vi "SPCC_Assignment_Server.vi"() -> ()   [LabVIEW 2023]
uses:
  LoginEnumStates.ctl
  <vilib>/Utility/file.llb/Write Delimited Spreadsheet (string).vi
  <vilib>/Utility/file.llb/Read Delimited Spreadsheet (string).vi
  <vilib>/regexp/Match Regular Expression.xnode
panel:
  in  "LoginUI":enum32{"Page 1"}(tab)
  in  "Password":string
  in  "User Name":string
  in  "btnLogin":bool
  in  "ZoneUI":enum32{"Page 1"}(tab)
  out "date/time string":string
  out "Alert":bool
  out "1T":bool caption="1A 3"
  out "1B":bool caption="1A 2"
  out "1A":bool
  out "Zone1":bool
  out "6T":bool caption="1A 3"
  out "6B":bool caption="1A 2"
  out "6A":bool caption="1A"
  out "Zone6":bool
  out "5T":bool caption="1A 3"
  out "5B":bool caption="1A 2"
  out "5A":bool caption="1A"
  out "Zone5":bool
  out "4T":bool caption="1A 3"
  out "4B":bool caption="1A 2"
  out "4A":bool caption="1A"
  out "Zone4":bool
  out "3T":bool caption="1A 3"
  out "3B":bool caption="1A 2"
  out "3A":bool caption="1A"
  out "Zone3":bool
  out "2T":bool caption="1A 3"
  out "2B":bool caption="1A 2"
  out "2A":bool caption="1A"
  out "Zone2":bool
  out "UserType":string
  in  "UserUi":enum32{"Page 1"}(tab)
  in  "btnUserEnd":bool
  in  "btnUserLogout":bool
  in  "AdminUI":enum32{"Page 2"}(tab)
  in  "btnViewLogs":bool
  in  "btnRegister":bool
  in  "btnAdminLogout":bool
  in  "btnAdminEnd":bool
  in  "User Table":string[][](table)
  in  "Tamper":cluster{u32, u32}[](array[cluster])
  in  "Bypass":cluster{u32, u32}[](array[cluster])
  in  "Alarm":cluster{u32, u32}[](array[cluster])
  in  "Normal":cluster{u32, u32}[](array[cluster])
  in  "ViewLogsUI":enum32{"Page 1"}(tab)
  in  "LogsTable":string[][](table)
  in  "btnMainMenu":bool
  # "LOGIN"
  # "Green   = Normal\nRed       = Alarm\nBlue      = Bypass\nOrange = Tamper"
  # "Zone Status Indicator"
  # "Zone 1"
  # "Alarm"
  # "Bypass"
  # "Tamper"
  # "Zone 6"
  # "Alarm"
  # "Bypass"
  # "Tamper"
  # "Zone 5"
  # "Alarm"
  # "Bypass"
  # "Tamper"
  # "Zone 4"
  # "Alarm"
  # "Bypass"
  # "Tamper"
  # "Zone 3"
  # "Alarm"
  # "Bypass"
  # "Tamper"
  # "Zone 2"
  # "Alarm"
  # "Bypass"
  # "Tamper"
  # "ADMIN MENU"
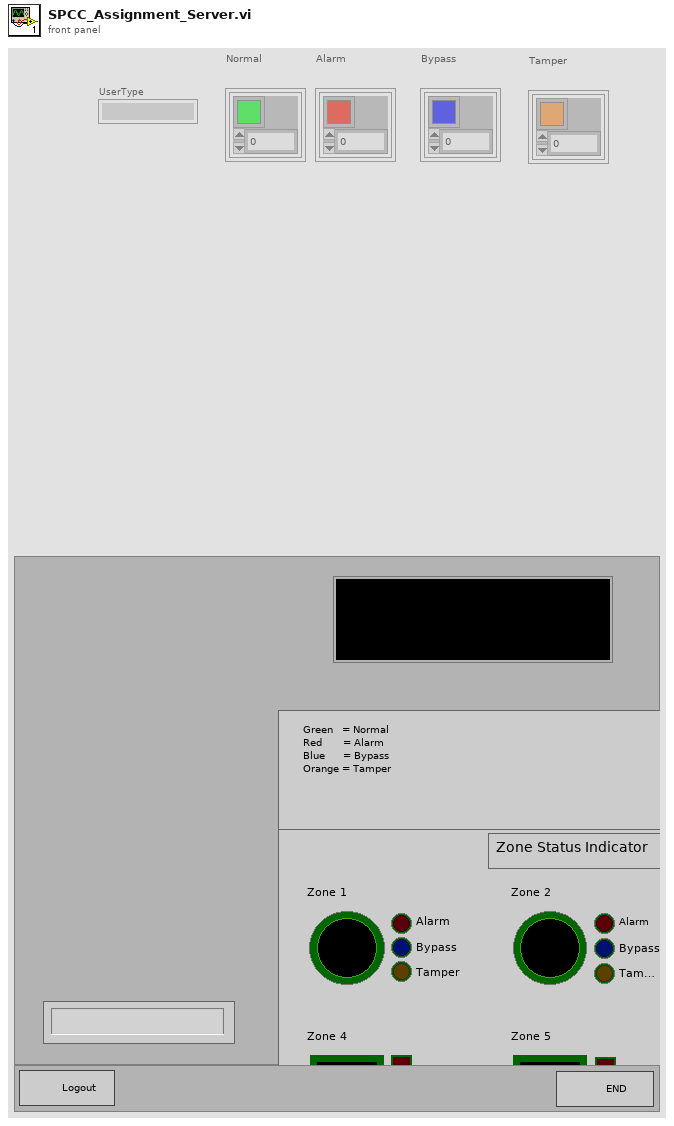
[diagram p1: front panel]
types:
  T1 = typedef "LoginEnumStates.ctl" = enum16{"Init", "Wait", "Login", "UIBuild", "Logout", "Register", "End"}
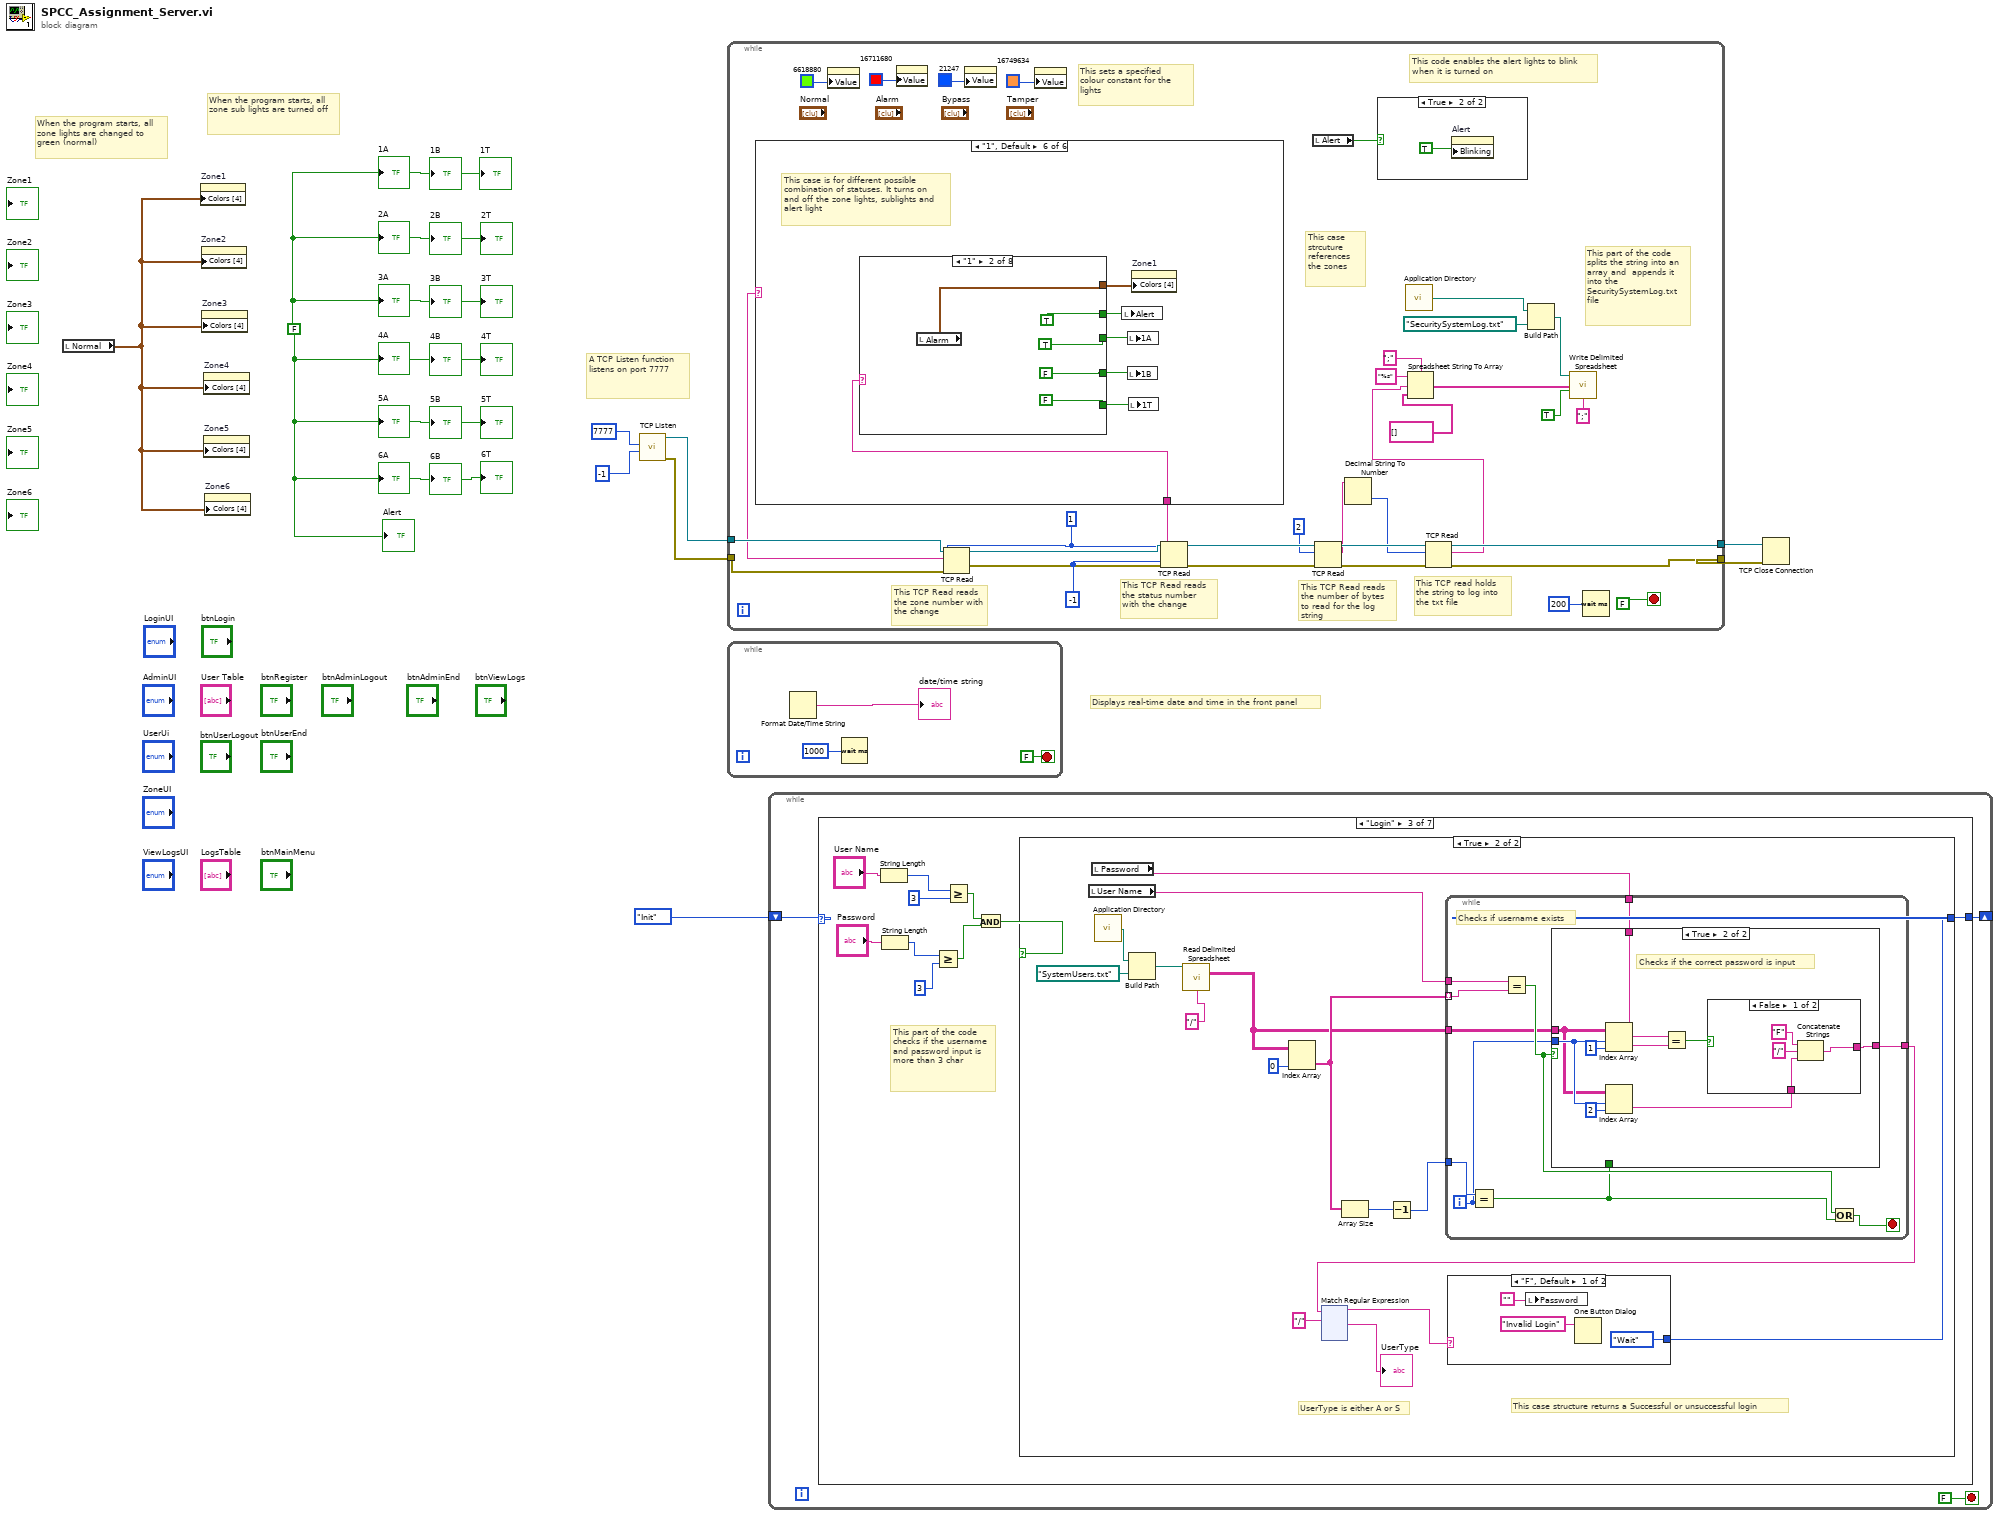
[diagram p0: block diagram]
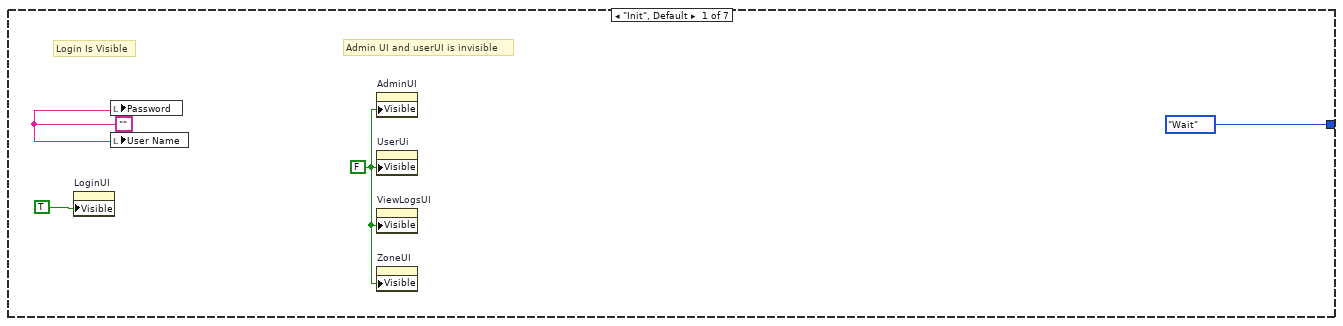
[diagram p2: hidden frame]
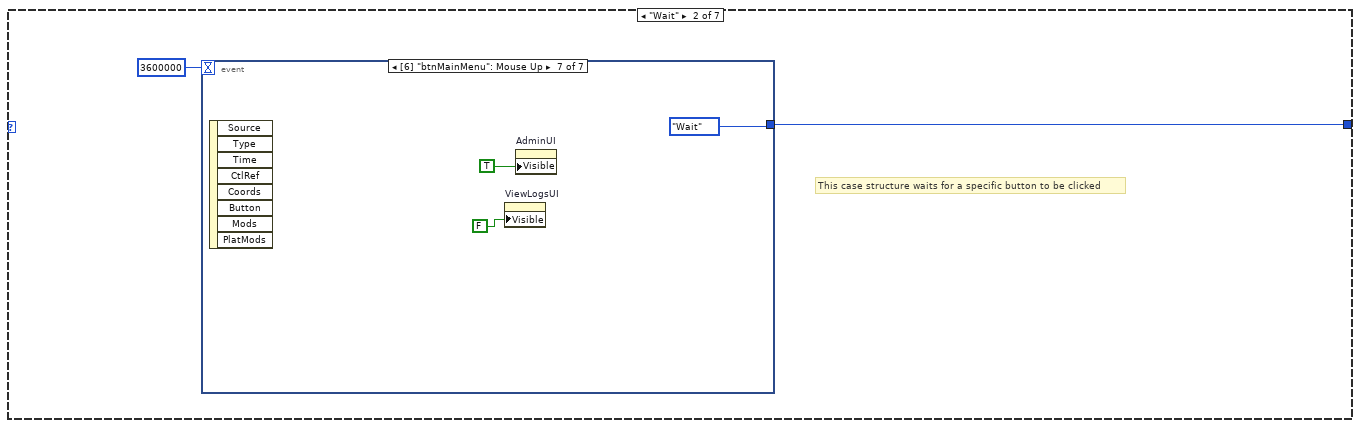
[diagram p3: hidden frame]
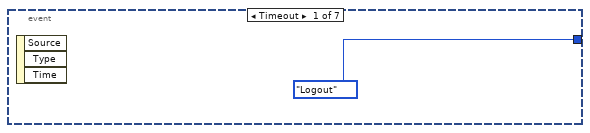
[diagram p4: hidden frame]
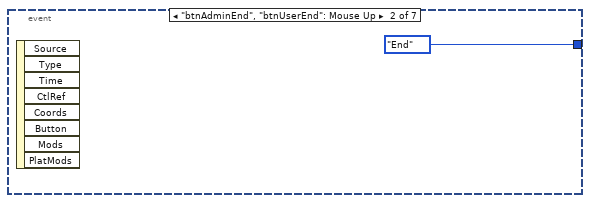
[diagram p5: hidden frame]
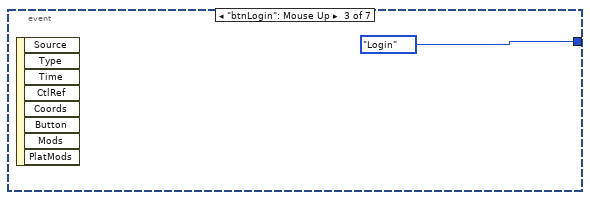
[diagram p6: hidden frame]
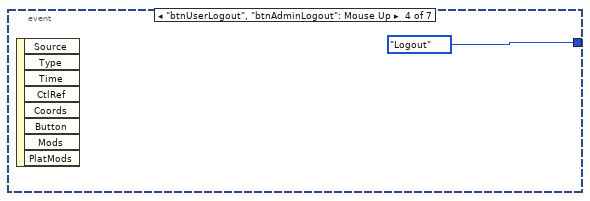
[diagram p7: hidden frame]
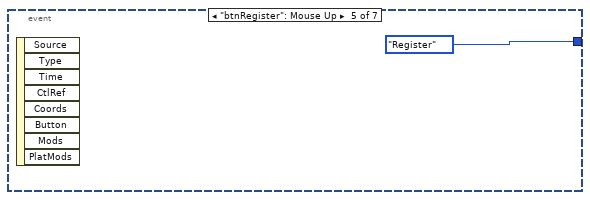
[diagram p8: hidden frame]
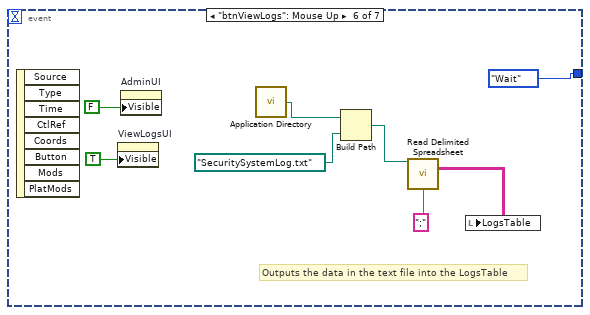
[diagram p9: hidden frame]
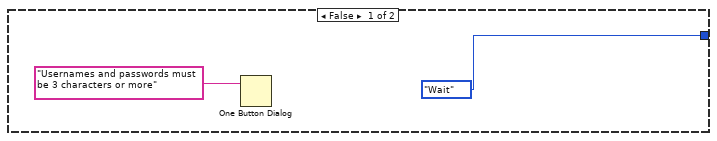
[diagram p10: hidden frame]
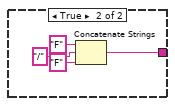
[diagram p12: hidden frame]
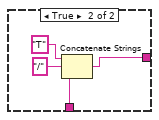
[diagram p13: hidden frame]
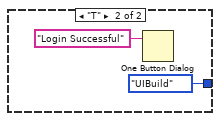
[diagram p14: hidden frame]
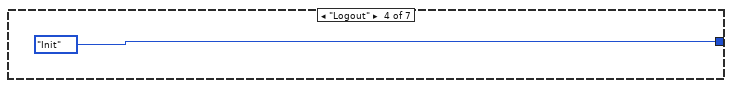
[diagram p15: hidden frame]
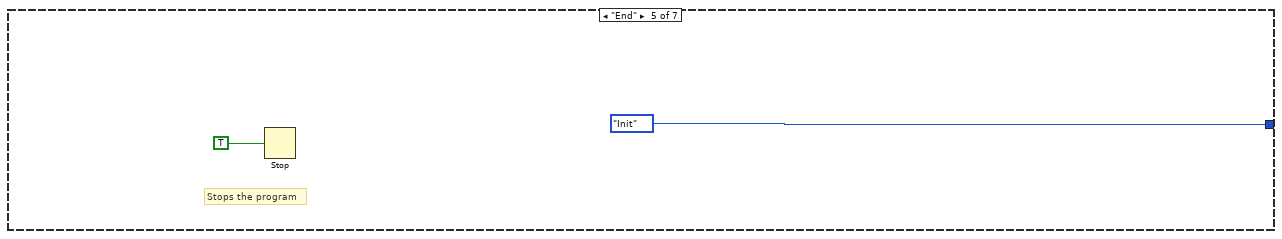
[diagram p16: hidden frame]
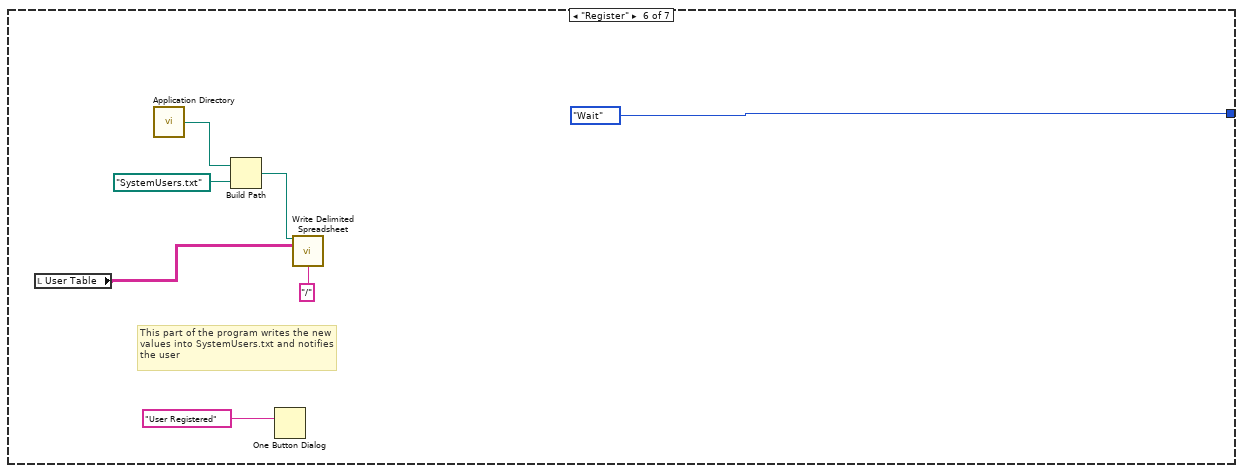
[diagram p17: hidden frame]
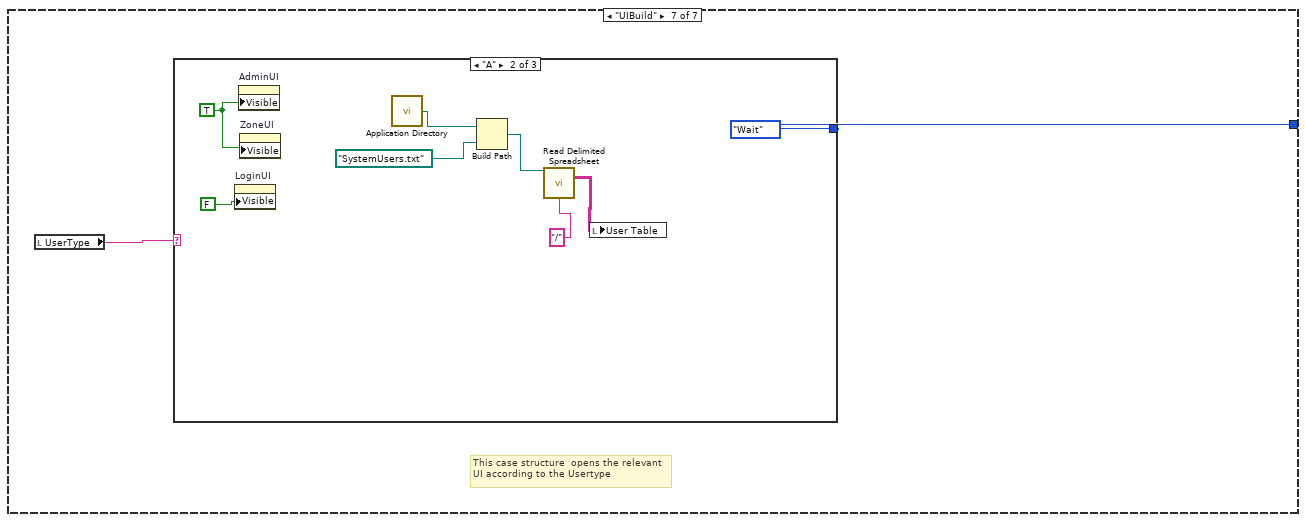
[diagram p18: hidden frame]
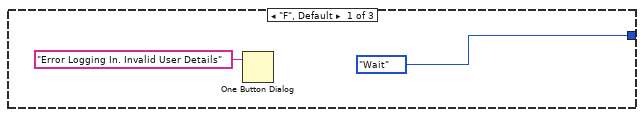
[diagram p19: hidden frame]
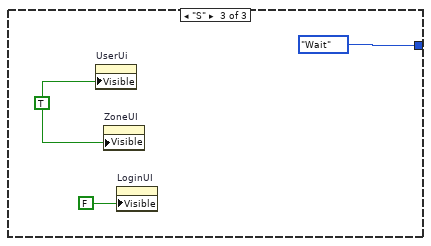
[diagram p20: hidden frame]
diagram:
  w2 = FALSE
  # "Displays real-time date and time in the front panel"
  # "A TCP Listen function listens on port 7777"
  # "When the program starts, all zone sub lights are turned off"
  # "When the program starts, all zone lights are changed to green (normal)"
  n1 = local read "Normal"() -> (w3:cluster{u32, u32}[])
  n2 = property on="Zone1" class="Bool (strict)"("Colors [4]"=w3) -> ()  [unwired: 2 in, 2 out]
  n3 = property on="Zone2" class="Bool (strict)"("Colors [4]"=w3) -> ()  [unwired: 2 in, 2 out]
  n4 = property on="Zone3" class="Bool (strict)"("Colors [4]"=w3) -> ()  [unwired: 2 in, 2 out]
  n5 = property on="Zone4" class="Bool (strict)"("Colors [4]"=w3) -> ()  [unwired: 2 in, 2 out]
  n6 = property on="Zone5" class="Bool (strict)"("Colors [4]"=w3) -> ()  [unwired: 2 in, 2 out]
  n7 = property on="Zone6" class="Bool (strict)"("Colors [4]"=w3) -> ()  [unwired: 2 in, 2 out]
  n8 = call <vilib>:"TCP Listen.vi"("timeout ms (wait forever: -1)"=-1, "port"=u16 7777) -> ("error out"=w7:errorcluster, "connection ID"=w9:refnum<k5>)  [unwired: 5 in, 3 out]
  n9 = while {
    tunnel: w9 -> [w42]
    tunnel: [w30] -> w8
    tunnel: w7 -> [w40]
    tunnel: [w29] -> w6
    stop <- FALSE stop-if-true
    w37 = -1 ("timeout ms (25000)")
    w38 = 1 ("bytes to read")
    # "This case strcuture references the zones"
    # "This sets a specified colour constant for the lights"
    # "This code enables the alert lights to blink when it is turned on"
    # "This part of the code splits the string into an array and  appends it into the SecuritySystemLog.txt file"
    # "This TCP read holds the string to log into the txt file"
    # "This TCP Read reads the number of bytes to read for the log string"
    # "This TCP Read reads the status number with the change"
    # "This TCP Read reads the zone number with the change"
    n10 = property class="ColBox"("Value"=u32 6618880) -> ()  [unwired: 2 in, 2 out]
    n11 = property class="ColBox"("Value"=u32 16711680) -> ()  [unwired: 2 in, 2 out]
    n12 = TCP Read(connection ID=w42, bytes to read=w38, error in (no error)=w40, 9:w37) -> (connection ID out=w41:refnum<k5>, data out=w36:string, error out=w39:errorcluster)  [unwired: 1 in]
    n13 = property class="ColBox"("Value"=u32 21247) -> ()  [unwired: 2 in, 2 out]
    n14 = property class="ColBox"("Value"=u32 16749634) -> ()  [unwired: 2 in, 2 out]
    n15 = TCP Read(connection ID=w41, bytes to read=w38, error in (no error)=w39, 9:w37) -> (connection ID out=w17:refnum<k5>, data out=w43:string, error out=w16:errorcluster)  [unwired: 1 in]
    n16 = case shown="\"1\", Default" w36 {
      tunnel: w43 -> [w51 w90 w131 w171 w210 w251]
      frame "2" {
        # "This case is for different possible combination of statuses. It turns on and off the zone lights, sublights and alert light"
        n17 = case shown="\"0\", Default" w51 {
          tunnel: [w53 w58 w63 w68 w73 w78 w83 w85] -> w50
          tunnel: [w52 TRUE FALSE TRUE FALSE TRUE FALSE w84] -> w49
          tunnel: [w52 FALSE TRUE TRUE FALSE FALSE TRUE w84] -> w48
          tunnel: [w52 FALSE FALSE FALSE TRUE TRUE TRUE w84] -> w47
          tunnel: [w52 TRUE FALSE FALSE TRUE TRUE TRUE w84] -> w46
          frame "0", Default {
            w52 = FALSE
            n18 = local read "Normal"() -> (w53:cluster{u32, u32}[])
          }
          frame "1" {
            n19 = local read "Alarm"() -> (w58:cluster{u32, u32}[])
          }
          frame "2" {
            n20 = local read "Bypass"() -> (w63:cluster{u32, u32}[])
          }
          frame "3" {
            n21 = local read "Bypass"() -> (w68:cluster{u32, u32}[])
          }
          frame "4" {
            n22 = local read "Tamper"() -> (w73:cluster{u32, u32}[])
          }
          frame "5" {
            n23 = local read "Tamper"() -> (w78:cluster{u32, u32}[])
          }
          frame "6" {
            n24 = local read "Tamper"() -> (w83:cluster{u32, u32}[])
          }
          frame "7" {
            w84 = TRUE
            n25 = local read "Tamper"() -> (w85:cluster{u32, u32}[])
          }
        }
        n26 = local write "Alert"(w46) -> ()
        n27 = local write "2A"(w49) -> ()
        n28 = local write "2B"(w48) -> ()
        n29 = local write "2T"(w47) -> ()
        n30 = property on="Zone2" class="Bool (strict)"("Colors [4]"=w50) -> ()  [unwired: 2 in, 2 out]
      }
      frame "3" {
        # "This case is for different possible combination of statuses. It turns on and off the zone lights, sublights and alert light"
        n31 = case shown="\"7\"" w90 {
          tunnel: [w93 w98 w103 w108 w113 w118 w123 w125] -> w91
          tunnel: [w92 TRUE FALSE TRUE FALSE TRUE FALSE w124] -> w89
          tunnel: [w92 FALSE TRUE TRUE FALSE FALSE TRUE w124] -> w88
          tunnel: [w92 FALSE FALSE FALSE TRUE TRUE TRUE w124] -> w87
          tunnel: [w92 TRUE FALSE FALSE TRUE TRUE TRUE w124] -> w86
          frame "0", Default {
            w92 = FALSE
            n32 = local read "Normal"() -> (w93:cluster{u32, u32}[])
          }
          frame "1" {
            n33 = local read "Alarm"() -> (w98:cluster{u32, u32}[])
          }
          frame "2" {
            n34 = local read "Bypass"() -> (w103:cluster{u32, u32}[])
          }
          frame "3" {
            n35 = local read "Bypass"() -> (w108:cluster{u32, u32}[])
          }
          frame "4" {
            n36 = local read "Tamper"() -> (w113:cluster{u32, u32}[])
          }
          frame "5" {
            n37 = local read "Tamper"() -> (w118:cluster{u32, u32}[])
          }
          frame "6" {
            n38 = local read "Tamper"() -> (w123:cluster{u32, u32}[])
          }
          frame "7" {
            w124 = TRUE
            n39 = local read "Tamper"() -> (w125:cluster{u32, u32}[])
          }
        }
        n40 = local write "Alert"(w86) -> ()
        n41 = local write "3A"(w89) -> ()
        n42 = local write "3B"(w88) -> ()
        n43 = local write "3T"(w87) -> ()
        n44 = property on="Zone3" class="Bool (strict)"("Colors [4]"=w91) -> ()  [unwired: 2 in, 2 out]
      }
      frame "4" {
        # "This case is for different possible combination of statuses. It turns on and off the zone lights, sublights and alert light"
        n45 = case shown="\"7\"" w131 {
          tunnel: [w133 w138 w143 w148 w153 w158 w163 w165] -> w130
          tunnel: [w132 TRUE FALSE TRUE FALSE TRUE FALSE w164] -> w129
          tunnel: [w132 FALSE FALSE FALSE TRUE TRUE TRUE w164] -> w128
          tunnel: [w132 FALSE TRUE TRUE FALSE FALSE TRUE w164] -> w127
          tunnel: [w132 TRUE FALSE FALSE TRUE TRUE TRUE w164] -> w126
          frame "0", Default {
            w132 = FALSE
            n46 = local read "Normal"() -> (w133:cluster{u32, u32}[])
          }
          frame "1" {
            n47 = local read "Alarm"() -> (w138:cluster{u32, u32}[])
          }
          frame "2" {
            n48 = local read "Bypass"() -> (w143:cluster{u32, u32}[])
          }
          frame "3" {
            n49 = local read "Bypass"() -> (w148:cluster{u32, u32}[])
          }
          frame "4" {
            n50 = local read "Tamper"() -> (w153:cluster{u32, u32}[])
          }
          frame "5" {
            n51 = local read "Tamper"() -> (w158:cluster{u32, u32}[])
          }
          frame "6" {
            n52 = local read "Tamper"() -> (w163:cluster{u32, u32}[])
          }
          frame "7" {
            w164 = TRUE
            n53 = local read "Tamper"() -> (w165:cluster{u32, u32}[])
          }
        }
        n54 = local write "4A"(w129) -> ()
        n55 = local write "4B"(w127) -> ()
        n56 = local write "4T"(w128) -> ()
        n57 = local write "Alert"(w126) -> ()
        n58 = property on="Zone4" class="Bool (strict)"("Colors [4]"=w130) -> ()  [unwired: 2 in, 2 out]
      }
      frame "5" {
        # "This case is for different possible combination of statuses. It turns on and off the zone lights, sublights and alert light"
        n59 = case shown="\"0\", Default" w171 {
          tunnel: [w173 w178 w183 w188 w193 w198 w203 w205] -> w170
          tunnel: [w172 TRUE FALSE TRUE FALSE TRUE FALSE w204] -> w169
          tunnel: [w172 FALSE FALSE FALSE TRUE TRUE TRUE w204] -> w168
          tunnel: [w172 FALSE TRUE TRUE FALSE FALSE TRUE w204] -> w167
          tunnel: [w172 TRUE FALSE FALSE TRUE TRUE TRUE w204] -> w166
          frame "0", Default {
            w172 = FALSE
            n60 = local read "Normal"() -> (w173:cluster{u32, u32}[])
          }
          frame "1" {
            n61 = local read "Alarm"() -> (w178:cluster{u32, u32}[])
          }
          frame "2" {
            n62 = local read "Bypass"() -> (w183:cluster{u32, u32}[])
          }
          frame "3" {
            n63 = local read "Bypass"() -> (w188:cluster{u32, u32}[])
          }
          frame "4" {
            n64 = local read "Tamper"() -> (w193:cluster{u32, u32}[])
          }
          frame "5" {
            n65 = local read "Tamper"() -> (w198:cluster{u32, u32}[])
          }
          frame "6" {
            n66 = local read "Tamper"() -> (w203:cluster{u32, u32}[])
          }
          frame "7" {
            w204 = TRUE
            n67 = local read "Tamper"() -> (w205:cluster{u32, u32}[])
          }
        }
        n68 = local write "Alert"(w166) -> ()
        n69 = local write "5A"(w169) -> ()
        n70 = local write "5B"(w167) -> ()
        n71 = local write "5T"(w168) -> ()
        n72 = property on="Zone5" class="Bool (strict)"("Colors [4]"=w170) -> ()  [unwired: 2 in, 2 out]
      }
      frame "6" {
        # "This case is for different possible combination of statuses. It turns on and off the zone lights, sublights and alert light"
        n73 = case shown="\"0\", Default" w210 {
          tunnel: [w213 w218 w223 w228 w233 w238 w243 w245] -> w211
          tunnel: [w212 TRUE FALSE TRUE FALSE TRUE FALSE w244] -> w209
          tunnel: [w212 FALSE FALSE FALSE TRUE TRUE TRUE w244] -> w208
          tunnel: [w212 FALSE TRUE TRUE FALSE FALSE TRUE w244] -> w207
          tunnel: [w212 TRUE FALSE FALSE TRUE TRUE TRUE w244] -> w206
          frame "0", Default {
            w212 = FALSE
            n74 = local read "Normal"() -> (w213:cluster{u32, u32}[])
          }
          frame "1" {
            (unwired) TRUE
            n75 = local read "Alarm"() -> (w218:cluster{u32, u32}[])
          }
          frame "2" {
            (unwired) TRUE
            n76 = local read "Bypass"() -> (w223:cluster{u32, u32}[])
          }
          frame "3" {
            (unwired) TRUE
            n77 = local read "Bypass"() -> (w228:cluster{u32, u32}[])
          }
          frame "4" {
            (unwired) TRUE
            n78 = local read "Tamper"() -> (w233:cluster{u32, u32}[])
          }
          frame "5" {
            (unwired) TRUE
            n79 = local read "Tamper"() -> (w238:cluster{u32, u32}[])
          }
          frame "6" {
            (unwired) TRUE
            n80 = local read "Tamper"() -> (w243:cluster{u32, u32}[])
          }
          frame "7" {
            w244 = TRUE
            n81 = local read "Tamper"() -> (w245:cluster{u32, u32}[])
          }
        }
        n82 = local write "Alert"(w206) -> ()
        n83 = local write "6A"(w209) -> ()
        n84 = local write "6B"(w207) -> ()
        n85 = local write "6T"(w208) -> ()
        n86 = property on="Zone6" class="Bool (strict)"("Colors [4]"=w211) -> ()  [unwired: 2 in, 2 out]
      }
      frame "1", Default {
        # "This case is for different possible combination of statuses. It turns on and off the zone lights, sublights and alert light"
        n87 = case shown="\"1\"" w251 {
          tunnel: [w253 w258 w263 w268 w273 w278 w283 w285] -> w250
          tunnel: [w252 TRUE FALSE TRUE FALSE TRUE FALSE w284] -> w249
          tunnel: [w252 FALSE TRUE TRUE FALSE FALSE TRUE w284] -> w248
          tunnel: [w252 FALSE FALSE FALSE TRUE TRUE TRUE w284] -> w247
          tunnel: [w252 TRUE FALSE FALSE TRUE TRUE TRUE w284] -> w246
          frame "0", Default {
            w252 = FALSE
            n88 = local read "Normal"() -> (w253:cluster{u32, u32}[])
          }
          frame "1" {
            n89 = local read "Alarm"() -> (w258:cluster{u32, u32}[])
          }
          frame "2" {
            n90 = local read "Bypass"() -> (w263:cluster{u32, u32}[])
          }
          frame "3" {
            n91 = local read "Bypass"() -> (w268:cluster{u32, u32}[])
          }
          frame "4" {
            n92 = local read "Tamper"() -> (w273:cluster{u32, u32}[])
          }
          frame "5" {
            n93 = local read "Tamper"() -> (w278:cluster{u32, u32}[])
          }
          frame "6" {
            n94 = local read "Tamper"() -> (w283:cluster{u32, u32}[])
          }
          frame "7" {
            w284 = TRUE
            n95 = local read "Tamper"() -> (w285:cluster{u32, u32}[])
          }
        }
        n96 = local write "Alert"(w246) -> ()
        n97 = local write "1A"(w249) -> ()
        n98 = local write "1B"(w248) -> ()
        n99 = local write "1T"(w247) -> ()
        n100 = property on="Zone1" class="Bool (strict)"("Colors [4]"=w250) -> ()  [unwired: 2 in, 2 out]
      }
    }
    n101 = local read "Alert"() -> (w10:bool)
    n102 = TCP Read(connection ID=w17, bytes to read=2, error in (no error)=w16) -> (connection ID out=w15:refnum<k5>, data out=w12:string, error out=w14:errorcluster)  [unwired: 2 in]
    n103 = Decimal String To Number(string=w12) -> (number=w11:i32)  [unwired: 2 in, 1 out]
    n104 = case shown="True" w10 {
      frame False {
        n105 = property on="Alert" class="Bool (strict)"("Blinking"=FALSE) -> ()  [unwired: 2 in, 2 out]
      }
      frame True {
        n106 = property on="Alert" class="Bool (strict)"("Blinking"=TRUE) -> ()  [unwired: 2 in, 2 out]
      }
    }
    n107 = call <vilib>:"Application Directory.vi"() -> ("Application Directory"=w27:path)
    n108 = TCP Read(connection ID=w15, bytes to read=w11, error in (no error)=w14) -> (connection ID out=w30:refnum<k5>, data out=w24:string, error out=w29:errorcluster)  [unwired: 2 in]
    n109 = Spreadsheet String To Array(delimiter (Tab)=";", format string="%s", spreadsheet string=w24, array type (2D Dbl)=string[] []) -> (array=w18:string[])
    n110 = Build Path(base path=w27, name or relative path=path "SecuritySystemLog.txt") -> (appended path=w28:path)
    n111 = call-poly <vilib>:"Write Delimited Spreadsheet.vi"("file path (dialog if empty)"=w28, "1D data"=w18, "append to file? (new file:F)"=TRUE, "delimiter (\\t)"=";" ("delimiter (\\t)")) -> ()  [unwired: 10 in, 2 out]
    n112 = Wait (ms)(milliseconds to wait=u32 200) -> ()  [unwired: 1 out]
  }
  n113 = while {
    stop <- FALSE stop-if-true
    n114 = Format Date/Time String() -> (date/time string=→"date/time string":string)  [unwired: 3 in]
    n115 = Wait (ms)(milliseconds to wait=u32 1000) -> ()  [unwired: 1 out]
  }
  n116 = while {
    shift-right: [w290] -> _
    shift-left: LoginEnumStates."Init" -> [w291]
    stop <- FALSE stop-if-true
    n117 = case shown="\"Login\"" w291 {
      tunnel: [LoginEnumStates."Wait" w296 w322 LoginEnumStates."Init" LoginEnumStates."Init" LoginEnumStates."Wait" w508] -> w290
      frame "Init", Default {
        w292 = FALSE ("Visible")
        w294 = ""
        # "Admin UI and userUI is invisible"
        # "Login Is Visible"
        n118 = property on="LoginUI" class="TabCtl (strict)"("Visible"=TRUE) -> ()  [unwired: 2 in, 2 out]
        n119 = local write "Password"(w294) -> ()
        n120 = local write "User Name"(w294) -> ()
        n121 = property on="AdminUI" class="TabCtl (strict)"("Visible"=w292) -> ()  [unwired: 2 in, 2 out]
        n122 = property on="UserUi" class="TabCtl (strict)"("Visible"=w292) -> ()  [unwired: 2 in, 2 out]
        n123 = property on="ViewLogsUI" class="TabCtl (strict)"("Visible"=w292) -> ()  [unwired: 2 in, 2 out]
        n124 = property on="ZoneUI" class="TabCtl (strict)"("Visible"=w292) -> ()  [unwired: 2 in, 2 out]
      }
      frame "Wait" {
        # "This case structure waits for a specific button to be clicked"
        n125 = event shown="[6] \"btnMainMenu\": Mouse Up" {
          selector: _ -> [_ _ _ _ _ _ _]
          dyn-events: _ -> [_ _ _ _ _ _ _]
          timeout: 3600000 -> [_ _ _ _ _ _ _]
          tunnel: [LoginEnumStates."Logout" LoginEnumStates."End" LoginEnumStates."Login" LoginEnumStates."Logout" LoginEnumStates."Register" LoginEnumStates."Wait" LoginEnumStates."Wait"] -> w296
          event Timeout {
            n126 = event-data() -> ()  [unwired: 1 in, 3 out]
          }
          event "btnAdminEnd", "btnUserEnd": Mouse Up {
            n127 = event-data() -> ()  [unwired: 1 in, 8 out]
          }
          event "btnLogin": Mouse Up {
            n128 = event-data() -> ()  [unwired: 1 in, 8 out]
          }
          event "btnUserLogout", "btnAdminLogout": Mouse Up {
            n129 = event-data() -> ()  [unwired: 1 in, 8 out]
          }
          event "btnRegister": Mouse Up {
            n130 = event-data() -> ()  [unwired: 1 in, 8 out]
          }
          event "btnViewLogs": Mouse Up {
            # "Outputs the data in the text file into the LogsTable"
            n131 = event-data() -> ()  [unwired: 1 in, 8 out]
            n132 = property on="ViewLogsUI" class="TabCtl (strict)"("Visible"=TRUE) -> ()  [unwired: 2 in, 2 out]
            n133 = property on="AdminUI" class="TabCtl (strict)"("Visible"=FALSE) -> ()  [unwired: 2 in, 2 out]
            n134 = call <vilib>:"Application Directory.vi"() -> ("Application Directory"=w309:path)
            n135 = Build Path(base path=w309, name or relative path=path "SecuritySystemLog.txt") -> (appended path=w308:path)
            n136 = call-poly <vilib>:"Read Delimited Spreadsheet.vi"("file path (dialog if empty)"=w308, "delimiter (\\t)"=";" ("delimiter (\\t)")) -> ("all rows"=w310:string[][])  [unwired: 8 in, 5 out]
            n137 = local write "LogsTable"(w310) -> ()
          }
          event "btnMainMenu": Mouse Up {
            n138 = event-data() -> ()  [unwired: 1 in, 8 out]
            n139 = property on="ViewLogsUI" class="TabCtl (strict)"("Visible"=FALSE) -> ()  [unwired: 2 in, 2 out]
            n140 = property on="AdminUI" class="TabCtl (strict)"("Visible"=TRUE) -> ()  [unwired: 2 in, 2 out]
          }
        }
      }
      frame "Login" {
        # "This part of the code checks if the username and password input is more than 3 char"
        n141 = String Length(string="User Name") -> (length=w321:i32)
        n142 = String Length(string="Password") -> (length=w317:i32)
        n143 = Greater Or Equal?(x=w317, y=3) -> (x >= y?=w316:bool)
        n144 = Greater Or Equal?(x=w321, y=3) -> (x >= y?=w319:bool)
        n145 = And(x=w319, y=w316) -> (x .and. y?=w323:bool)
        n146 = case shown="True" w323 {
          tunnel: [LoginEnumStates."Wait" w341] -> w322
          frame False {
            n147 = One Button Dialog(message="Usernames and passwords must be 3 characters or more") -> ()  [unwired: 1 in, 1 out]
          }
          frame True {
            # "UserType is either A or S"
            # "This case structure returns a Successful or unsuccessful login"
            n148 = local read "User Name"() -> (w330:string)
            n149 = local read "Password"() -> (w331:string)
            n150 = call <vilib>:"Application Directory.vi"() -> ("Application Directory"=w340:path)
            n151 = Build Path(base path=w340, name or relative path=path "SystemUsers.txt") -> (appended path=w338:path)
            n152 = call-poly <vilib>:"Read Delimited Spreadsheet.vi"("file path (dialog if empty)"=w338, "delimiter (\\t)"="/" ("delimiter (\\t)")) -> ("all rows"=w333:string[][])  [unwired: 8 in, 5 out]
            n153 = Index Array "Index Array"(array=w333, index (col)=0 ("disabled index (col)")) -> (element=w336:string[])  [unwired: 1 in]
            n154 = Array Size(array=w336) -> (size(s)=w335:i32)
            n155 = Decrement(x=w335) -> (x-1=w334:i32)
            n156 = while {
              tunnel: w336 -> [w465] mode=indexing
              tunnel: w334 -> [w468]
              tunnel: w330 -> [w466]
              tunnel: w333 -> [w463]
              tunnel: w331 -> [w461]
              tunnel: [w460] -> w326
              i -> [w462]
              stop <- w467 stop-if-true
              # "Checks if username exists"
              n157 = Equal?(x=w468, y=w462) -> (x = y?=w459:bool)
              n158 = Equal?(x=w466, y=w465) -> (x = y?=w464:bool)
              n159 = case shown="True" w464 {
                tunnel: w463 -> [_ w479]
                tunnel: w462 -> [_ w481]
                tunnel: w461 -> [_ w483]
                tunnel: [w469 w478] -> w460
                tunnel: w459 -> [w470 _]
                frame False {
                  n160 = case shown="False" w470 {
                    tunnel: [_ w471] -> w469
                    frame False {
                    }
                    frame True {
                      n161 = Concatenate Strings("F" ("string"), "/" ("string"), "F" ("string")) -> (w471:string)
                    }
                  }
                }
                frame True {
                  # "Checks if the correct password is input"
                  n162 = Index Array "Index Array"(array=w479, index (row)=w481, index (col)=1) -> (element=w482:string)
                  n163 = Index Array "Index Array"(array=w479, index (row)=w481, index (col)=2) -> (element=w480:string)
                  n164 = Equal?(x=w483, y=w482) -> (x = y?=w475:bool)
                  n165 = case shown="False" w475 {
                    tunnel: w480 -> [w485 w489]
                    tunnel: [w484 w488] -> w478
                    frame False {
                      n166 = Concatenate Strings("F" ("string"), "/" ("string"), w485) -> (w484:string)
                    }
                    frame True {
                      n167 = Concatenate Strings("T" ("string"), "/" ("string"), w489) -> (w488:string)
                    }
                  }
                }
              }
              n168 = Or(x=w464, y=w459) -> (x .or. y?=w467:bool)
            }
            n169 = xnode "Match Regular Expression"("input string"=w326, "regular expression"="/") -> ("before match"=w328:string, "after match"=→"UserType":string)  [unwired: 4 in, 3 out]
            n170 = case shown="\"F\", Default" w328 {
              tunnel: [LoginEnumStates."Wait" LoginEnumStates."UIBuild"] -> w341
              frame "F", Default {
                n171 = local write "Password"("") -> ()
                n172 = One Button Dialog(message="Invalid Login") -> ()  [unwired: 1 in, 1 out]
              }
              frame "T" {
                n173 = One Button Dialog(message="Login Successful") -> ()  [unwired: 1 in, 1 out]
              }
            }
          }
        }
      }
      frame "Logout" {
      }
      frame "End" {
        # "Stops the program"
        n174 = Stop(stop? (T)=TRUE) -> ()
      }
      frame "Register" {
        # "This part of the program writes the new values into SystemUsers.txt and notifies the user"
        n175 = local read "User Table"() -> (w502:string[][])
        n176 = call <vilib>:"Application Directory.vi"() -> ("Application Directory"=w506:path)
        n177 = Build Path(base path=w506, name or relative path=path "SystemUsers.txt") -> (appended path=w504:path)
        n178 = One Button Dialog(message="User Registered") -> ()  [unwired: 1 in, 1 out]
        n179 = call-poly <vilib>:"Write Delimited Spreadsheet.vi"("file path (dialog if empty)"=w504, "2D data"=w502, "delimiter (\\t)"="/" ("delimiter (\\t)")) -> ()  [unwired: 11 in, 2 out]
      }
      frame "UIBuild" {
        # "This case structure  opens the relevant UI according to the Usertype"
        n180 = local read "UserType"() -> (w507:string)
        n181 = case shown="\"A\"" w507 {
          tunnel: [LoginEnumStates."Wait" LoginEnumStates."Wait" LoginEnumStates."Wait"] -> w508
          frame "F", Default {
            n182 = One Button Dialog(message="Error Logging In. Invalid User Details") -> ()  [unwired: 1 in, 1 out]
          }
          frame "A" {
            w513 = TRUE ("Visible")
            n183 = property on="LoginUI" class="TabCtl (strict)"("Visible"=FALSE) -> ()  [unwired: 2 in, 2 out]
            n184 = property on="AdminUI" class="TabCtl (strict)"("Visible"=w513) -> ()  [unwired: 2 in, 2 out]
            n185 = property on="ZoneUI" class="TabCtl (strict)"("Visible"=w513) -> ()  [unwired: 2 in, 2 out]
            n186 = call <vilib>:"Application Directory.vi"() -> ("Application Directory"=w517:path)
            n187 = Build Path(base path=w517, name or relative path=path "SystemUsers.txt") -> (appended path=w516:path)
            n188 = call-poly <vilib>:"Read Delimited Spreadsheet.vi"("file path (dialog if empty)"=w516, "delimiter (\\t)"="/" ("delimiter (\\t)")) -> ("all rows"=w512:string[][])  [unwired: 8 in, 5 out]
            n189 = local write "User Table"(w512) -> ()
          }
          frame "S" {
            w519 = TRUE ("Visible")
            n190 = property on="UserUi" class="TabCtl (strict)"("Visible"=w519) -> ()  [unwired: 2 in, 2 out]
            n191 = property on="ZoneUI" class="TabCtl (strict)"("Visible"=w519) -> ()  [unwired: 2 in, 2 out]
            n192 = property on="LoginUI" class="TabCtl (strict)"("Visible"=FALSE) -> ()  [unwired: 2 in, 2 out]
          }
        }
      }
    }
  }
  n193 = TCP Close Connection(connection ID=w8, error in (no error)=w6) -> ()  [unwired: 1 in, 2 out]
  "2A" <- w2
  "2B" <- w2
  "2T" <- w2
  "3A" <- w2
  "3B" <- w2
  "3T" <- w2
  "4A" <- w2
  "4B" <- w2
  "4T" <- w2
  "5A" <- w2
  "5B" <- w2
  "5T" <- w2
  "6A" <- w2
  "6B" <- w2
  "6T" <- w2
  "1A" <- w2
  "1B" <- w2
  "1T" <- w2
  "Alert" <- w2
